vi "XIPIN_QSGMII_3_3.vi"   [LabVIEW 2017]
doc: "The Xilinx Quad Serial Gigabit Media Independent Interface (QSGMII) LogiCORE provides a single lane high speed serial interface, operating at 5 Gigabits per second (Gbps) total throughput. The LogiCORE implements Cisco QSGMII V1.2 Specification. The core supports an optional serial MDIO management interface for accessing the internal management registers. The MDIO interface may be omitted to save slice logic, in which case a simplified management interface is provided via bit vectors. The core is designed to seamlessly interface with the Trimode Ethernet Media Access Controller (TEMAC) LogiCORE via the GMII. The QSGMII LogiCORE is available for the 7 Series, leveraging the capabilities of the embedded GT Transceivers in the device family.\n------------------------------------\n<b>Need License</b> : No"
uses:
  <vilib>/rvi/XilinxIP/XIPIN_XNode/niFpgaXIPIN.xnode
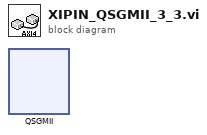
[diagram p0: block diagram]
diagram:
  n1 = xnode ("QSGMII")() -> ()
